vi "Subvi - marble identifier.vi"(11 "BrickReference in":T1) -> (2 "Array":dbl[](array[numeric]), 3 "BrickReference out":T1)   [LabVIEW 2016]
uses:
  <vilib>/NXT/Subs/LVHSConnector.ctl
  <vilib>/NXT/LegoClasses/BrickReference/BrickReference.lvclass
  <vilib>/NXT/Block Support/NXT_InputPort.ctl
  <vilib>/NXT/Dual Mode Library/Sensors/Touch_Pressed.vi
  <vilib>/NXT/Dual Mode Library/Sensors/EV3_Color_RGB.vi
  <vilib>/NXT/Dual Mode Library/prims/inRangeAndCoerce/inRangeAndCoerce_int.vi
  <vilib>/NXT/Dual Mode Library/Sensors/EV3_Color_Color.vi
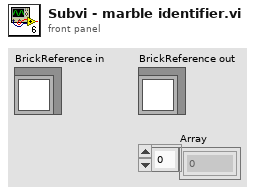
[diagram p1: front panel]
types:
  T1 = typedef "LVHSConnector.ctl" = refnum<class "BrickReference.lvclass">
  T2 = typedef "NXT_InputPort.ctl" = u32
  T3 = typedef "ColorSensorColors.ctl" = enum16{"No Color", "Black", "Blue", "Green", "Yellow", "Red", "White", "Brown"}
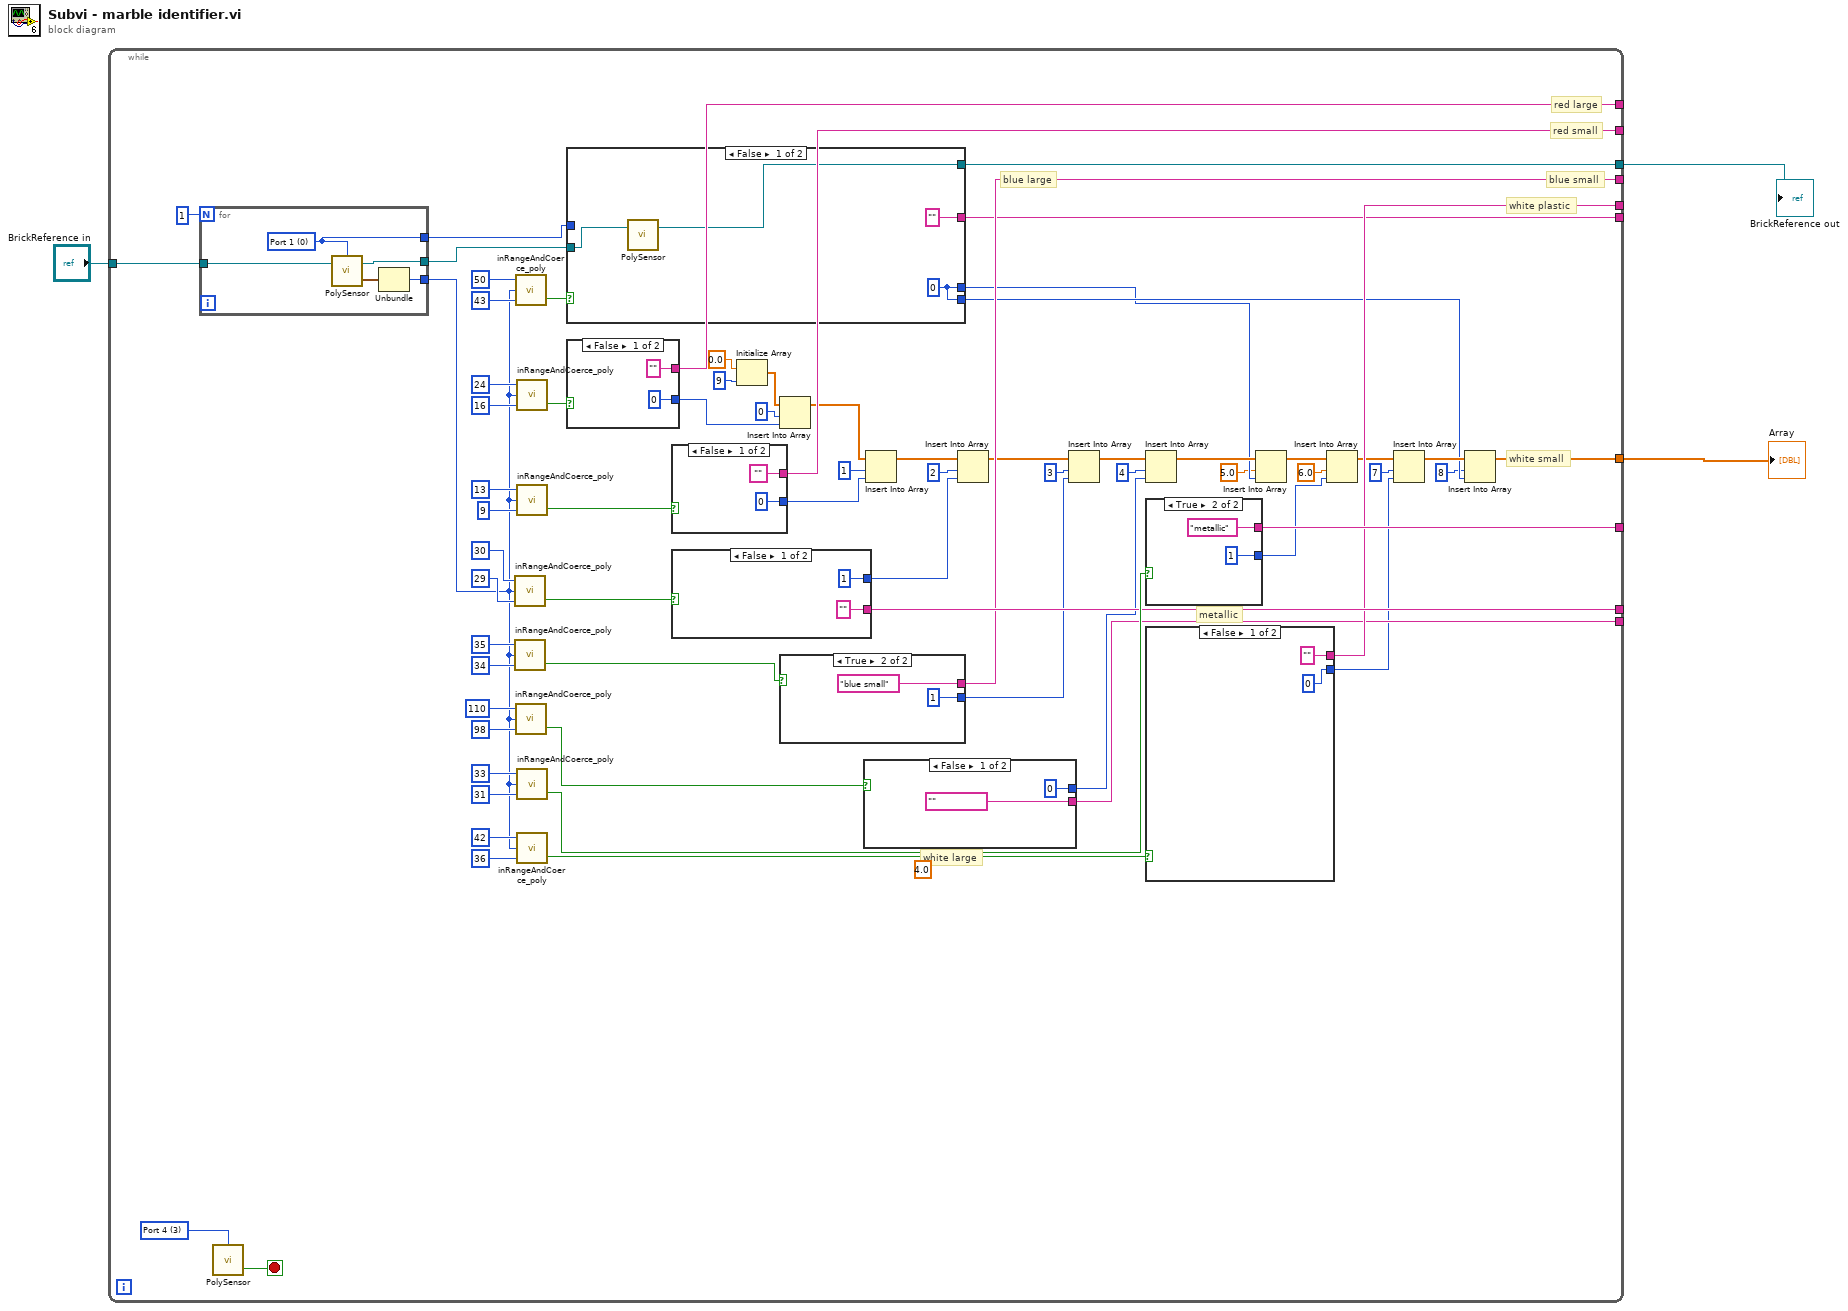
[diagram p0: block diagram]
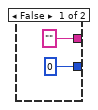
[diagram p2: hidden frame]
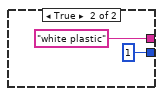
[diagram p3: hidden frame]
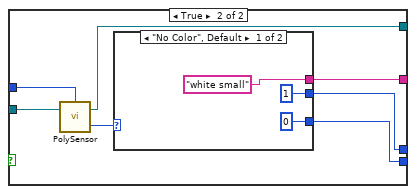
[diagram p4: hidden frame]
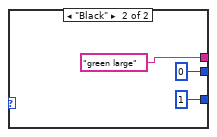
[diagram p5: hidden frame]
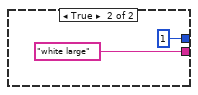
[diagram p6: hidden frame]
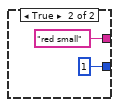
[diagram p7: hidden frame]
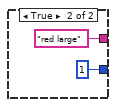
[diagram p8: hidden frame]
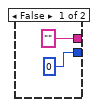
[diagram p9: hidden frame]
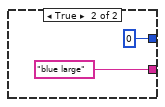
[diagram p10: hidden frame]
diagram:
  n1 = while {
    tunnel: "BrickReference in" -> [w49]
    tunnel: [w43] -> _
    tunnel: [w42] -> _
    tunnel: [w41] -> _
    tunnel: [w40] -> _
    tunnel: [w39] -> _
    tunnel: [w38] -> _
    tunnel: [w37] -> _
    tunnel: [w36] -> _
    tunnel: [w5] -> w2
    tunnel: [w4] -> w3
    stop <- w52 stop-if-true
    (unwired) sgl 4.0 ("Time (1 sec)")
    w51 = T2 3 items=["Port 1", "Port 2", "Port 3", "Port 4"] ("Port (Port 1)")
    # "metallic"
    # "white plastic"
    # "white small"
    # "white large"
    # "red small"
    # "red large"
    # "blue small"
    # "blue large"
    n2 = for {
      N: 1 -> [_]
      tunnel: w49 -> [w77]
      tunnel: [w76] -> w45
      tunnel: [w75] -> w35
      tunnel: [w74] -> w44
      w74 = T2 0 items=["Port 1", "Port 2", "Port 3", "Port 4"] ("Port (Port 1)")
      n3 = call-poly <vilib>:"PolySensor.vi"("NXT/EV3"=w77, "Port (Port 1)"=w74) -> ("RGB Color"=w78:cluster{"Red":u8, "Green":u8, "Blue":u8}, "NXT/EV3"=w75:T1)  [unwired: 1 in]
      n4 = Unbundle(w78) -> ("Green"=w76:u8)  [unwired: 2 out]
    }
    n5 = call-poly <vilib>:"PolySensor.vi"("Port (Port 1)"=w51) -> ("Yes / No"=w52:bool)  [unwired: 2 in, 1 out]
    n6 = call-poly <vilib>:"inRangeAndCoerce_poly.vi"("lower limit"=29, "x"=w45, "upper limit"=30) -> ("In Range?"=w60:bool)  [unwired: 1 out]
    n7 = call-poly <vilib>:"inRangeAndCoerce_poly.vi"("lower limit"=34, "x"=w45, "upper limit"=35) -> ("In Range?"=w59:bool)  [unwired: 1 out]
    n8 = call-poly <vilib>:"inRangeAndCoerce_poly.vi"("lower limit"=43, "x"=w45, "upper limit"=50) -> ("In Range?"=w55:bool)  [unwired: 1 out]
    n9 = call-poly <vilib>:"inRangeAndCoerce_poly.vi"("lower limit"=98, "x"=w45, "upper limit"=110) -> ("In Range?"=w56:bool)  [unwired: 1 out]
    n10 = call-poly <vilib>:"inRangeAndCoerce_poly.vi"("lower limit"=16, "x"=w45, "upper limit"=24) -> ("In Range?"=w58:bool)  [unwired: 1 out]
    n11 = call-poly <vilib>:"inRangeAndCoerce_poly.vi"("lower limit"=9, "x"=w45, "upper limit"=13) -> ("In Range?"=w57:bool)  [unwired: 1 out]
    n12 = call-poly <vilib>:"inRangeAndCoerce_poly.vi"("lower limit"=31, "x"=w45, "upper limit"=33) -> ("In Range?"=w46:bool)  [unwired: 1 out]
    n13 = call-poly <vilib>:"inRangeAndCoerce_poly.vi"("lower limit"=36, "x"=w45, "upper limit"=42) -> ("In Range?"=w54:bool)  [unwired: 1 out]
    n14 = case shown="False" w55 {
      tunnel: ["" w95] -> w37
      tunnel: w44 -> [_ w97]
      tunnel: w35 -> [w88 w94]
      tunnel: [w89 w93] -> w7
      tunnel: [w89 w92] -> w14
      tunnel: [w87 w91] -> w4
      frame False {
        w89 = 0
        n15 = call-poly <vilib>:"PolySensor.vi"("NXT/EV3"=w88) -> ("NXT/EV3"=w87:T1)  [unwired: 2 in, 1 out]
      }
      frame True {
        n16 = call-poly <vilib>:"PolySensor.vi"("NXT/EV3"=w94, "Port (Port 1)"=w97) -> ("Detected Color"=w96:T3, "NXT/EV3"=w91:T1)  [unwired: 1 in]
        n17 = case shown="\"No Color\", Default" w96 {
          tunnel: ["white small" "green large"] -> w95
          tunnel: [1 0] -> w93
          tunnel: [0 1] -> w92
          frame "No Color", Default {
          }
          frame "Black" {
          }
        }
      }
    }
    n18 = case shown="False" w58 {
      tunnel: ["" "red large"] -> w41
      tunnel: [0 1] -> w31
      frame False {
      }
      frame True {
      }
    }
    n19 = case shown="False" w57 {
      tunnel: ["" "red small"] -> w40
      tunnel: [0 1] -> w25
      frame False {
      }
      frame True {
      }
    }
    n20 = case shown="False" w60 {
      tunnel: ["" "blue large"] -> w43
      tunnel: [1 0] -> w26
      frame False {
      }
      frame True {
      }
    }
    n21 = Initialize Array(0.0 ("element"), 9 ("dimension size")) -> (w24:dbl[])
    n22 = Insert Into Array(array=w24, index=0, new element=w31) -> (w23:dbl[])
    n23 = case shown="True" w59 {
      tunnel: ["" "blue small"] -> w42
      tunnel: [0 1] -> w30
      frame False {
      }
      frame True {
      }
    }
    n24 = case shown="False" w56 {
      tunnel: ["" "white large"] -> w36
      tunnel: [0 1] -> w16
      frame False {
      }
      frame True {
      }
    }
    n25 = Insert Into Array(array=w23, index=1, new element=w25) -> (w22:dbl[])
    n26 = Insert Into Array(array=w22, index=2, new element=w26) -> (w21:dbl[])
    n27 = Insert Into Array(array=w21, index=3, new element=w30) -> (w20:dbl[])
    n28 = Insert Into Array(array=w20, index=4, new element=w16) -> (w10:dbl[])
    n29 = case shown="True" w46 {
      tunnel: ["" "metallic"] -> w39
      tunnel: [0 1] -> w8
      frame False {
      }
      frame True {
      }
    }
    n30 = case shown="False" w54 {
      tunnel: ["" "white plastic"] -> w38
      tunnel: [0 1] -> w13
      frame False {
      }
      frame True {
      }
    }
    n31 = Insert Into Array(array=w10, index=5.0 ("new element/subarray"), new element=w7) -> (w19:dbl[])
    n32 = Insert Into Array(array=w19, index=6.0 ("new element/subarray"), new element=w8) -> (w18:dbl[])
    n33 = Insert Into Array(array=w18, index=7, new element=w13) -> (w17:dbl[])
    n34 = Insert Into Array(array=w17, index=8, new element=w14) -> (w5:dbl[])
  }
  "BrickReference out" <- w3
  "Array" <- w2
